vi "Coil Test.vi"() -> ()   [LabVIEW 2025]
panel:
  in  "Pass Hipot Test":bool=TRUE
  in  "Coil Resistance":dbl
  in  "Stop":bool
  out "Results":string
  in  "Start":bool
  in  "Test Parameters":T1
  # "Simulated Coil Values"
  # "Ohms"
  # "Ohms"
  # "Ohms"
  # "Volts"
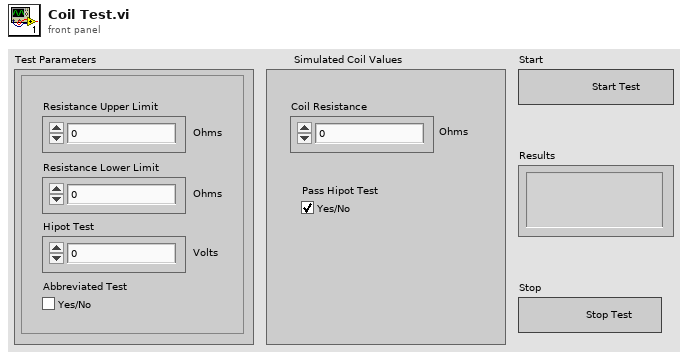
[diagram p1: front panel]
types:
  T1 = cluster{"Resistance Upper Limit":dbl, "Resistance Lower Limit ":dbl, "Hipot Test":dbl, "Abbreviated Test":bool}
  T2 = enum16{"Initialize", "Start", "Resistance Test", "Hipot Test", "Discard Coil", "Successful Coil", "Stop"}
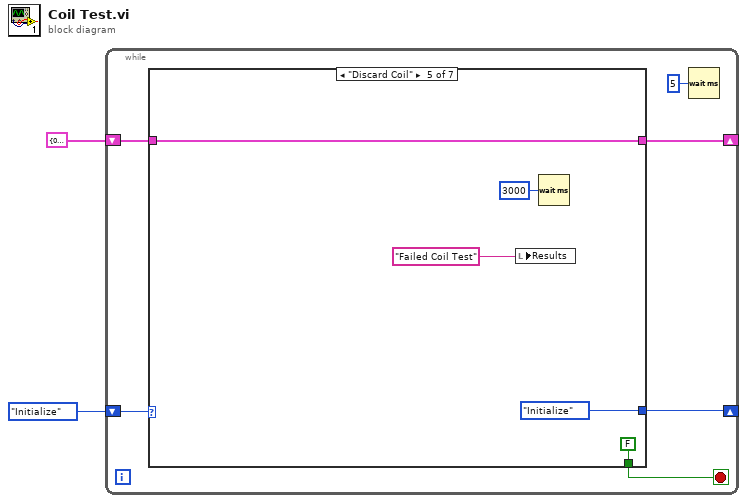
[diagram p0: block diagram]
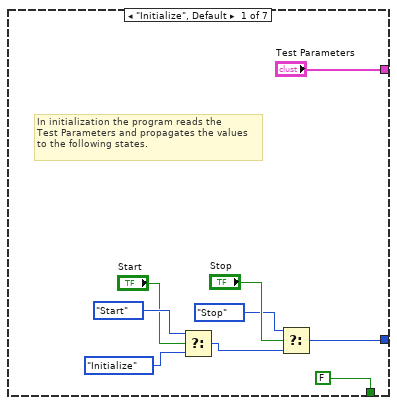
[diagram p2: hidden frame]
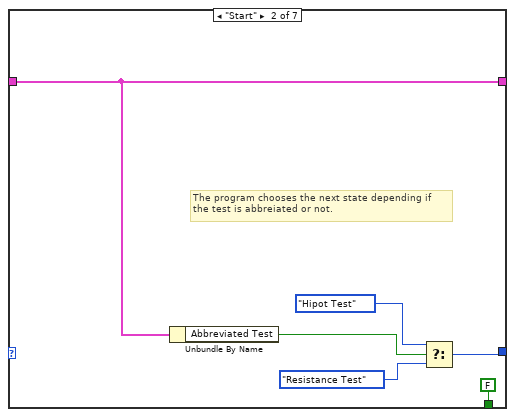
[diagram p3: hidden frame]
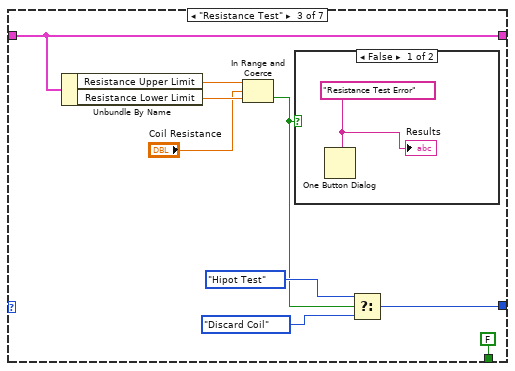
[diagram p4: hidden frame]
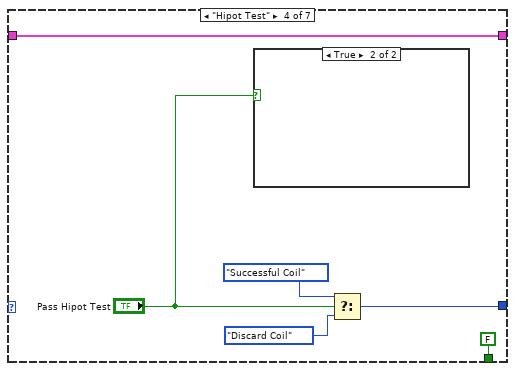
[diagram p6: hidden frame]
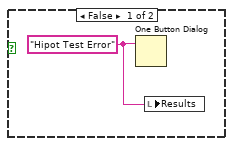
[diagram p7: hidden frame]
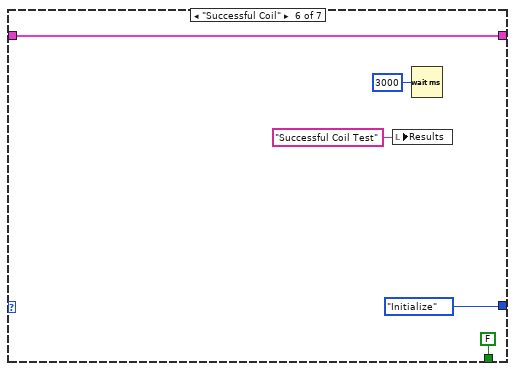
[diagram p8: hidden frame]
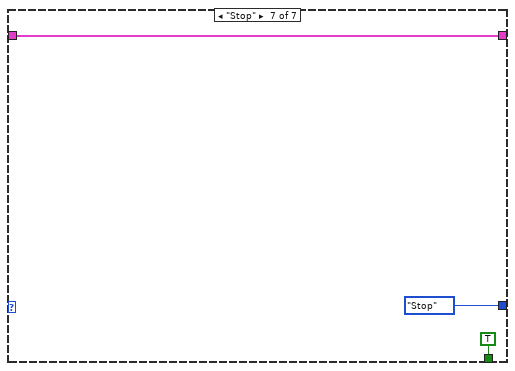
[diagram p9: hidden frame]
diagram:
  n1 = while {
    shift-right: [w5] -> _
    shift-left: T2."Initialize" -> [w8]
    shift-right: [w4] -> _
    shift-left: T1 {"Resistance Upper Limit"=0.0, "Resistance Lower Limit "=0.0, "Hipot Test"=0.0, "Abbreviated Test"=TRUE} ("Test Parameters") -> [w3]
    stop <- w6 stop-if-true
    n2 = case shown="\"Discard Coil\"" w8 {
      tunnel: [FALSE FALSE FALSE FALSE FALSE FALSE TRUE] -> w6
      tunnel: [w10 w18 w26 w37 T2."Initialize" T2."Initialize" T2."Stop"] -> w5
      tunnel: ["Test Parameters" w20 w32 w35 w45 w50 w53] -> w4
      tunnel: w3 -> [_ w20 w32 w35 w45 w50 w53]
      frame "Initialize", Default {
        # "In initialization the program reads the \nTest Parameters and propagates the values\nto the following states."
        n3 = Select(t=T2."Start", s="Start", f=T2."Initialize") -> (s? t:f=w12:T2)
        n4 = Select(t=T2."Stop", s="Stop", f=w12) -> (s? t:f=w10:T2)
      }
      frame "Start" {
        # "The program chooses the next state depending if\nthe test is abbreiated or not."
        n5 = Unbundle By Name(w20) -> ("Abbreviated Test"=w19:bool)
        n6 = Select(t=T2."Hipot Test", s=w19, f=T2."Resistance Test") -> (s? t:f=w18:T2)
      }
      frame "Resistance Test" {
        n7 = Unbundle By Name(w32) -> ("Resistance Upper Limit"=w31:dbl, "Resistance Lower Limit"=w30:dbl)
        n8 = In Range and Coerce(upper limit=w31, x="Coil Resistance", lower limit=w30) -> (In Range?=w25:bool)  [unwired: 1 out]
        n9 = case shown="False" w25 {
          frame False {
            w33 = "Resistance Test Error" ("message")
            n10 = One Button Dialog(message=w33) -> ()  [unwired: 1 in, 1 out]
            "Results" <- w33
          }
          frame True {
          }
        }
        n11 = Select(t=T2."Hipot Test", s=w25, f=T2."Discard Coil") -> (s? t:f=w26:T2)
      }
      frame "Hipot Test" {
        n12 = case shown="True" "Pass Hipot Test" {
          frame False {
            w40 = "Hipot Test Error"
            n13 = One Button Dialog(message=w40) -> ()  [unwired: 1 in, 1 out]
            n14 = local write "Results"(w40) -> ()
          }
          frame True {
          }
        }
        n15 = Select(t=T2."Successful Coil", s="Pass Hipot Test", f=T2."Discard Coil") -> (s? t:f=w37:T2)
      }
      frame "Discard Coil" {
        n16 = local write "Results"("Failed Coil Test" ("Results")) -> ()
        n17 = Wait (ms)(milliseconds to wait=u32 3000) -> ()  [unwired: 1 out]
      }
      frame "Successful Coil" {
        n18 = local write "Results"("Successful Coil Test" ("Results")) -> ()
        n19 = Wait (ms)(milliseconds to wait=u32 3000) -> ()  [unwired: 1 out]
      }
      frame "Stop" {
      }
    }
    n20 = Wait (ms)(milliseconds to wait=u32 5) -> ()  [unwired: 1 out]
  }
